vi "Msg Rescript.vi"() -> ()   [LabVIEW 2025]
uses:
  _Shared/Type.ctl
  _Shared/_Shared.lvlib
  _Msg Rescript/_Msg Rescript/_Msg Rescript.lvclass
  _Shared/Panel/Panel.lvlib
  _Shared/Tree/Tree.lvlib
  _Shared/Name Specs/Name Specs.lvclass
panel:
  out "Target":string
  in  "Tree":string(tree)
  in  "OK":bool
  # "Disclaimer: Please consider committing changes before AND after this action"
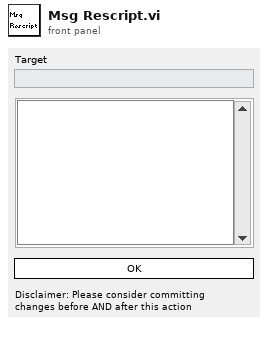
[diagram p1: front panel]
types:
  T1 = typedef "_Shared.lvlib/Type Name Library File Path.ctl" = map{T2, T3}
  T2 = typedef "_Shared.lvlib/Type.ctl" = enum16{"Actor", "Msg"}
  T3 = typedef "_Shared.lvlib/Name Library File Path.ctl" = map{string, path}
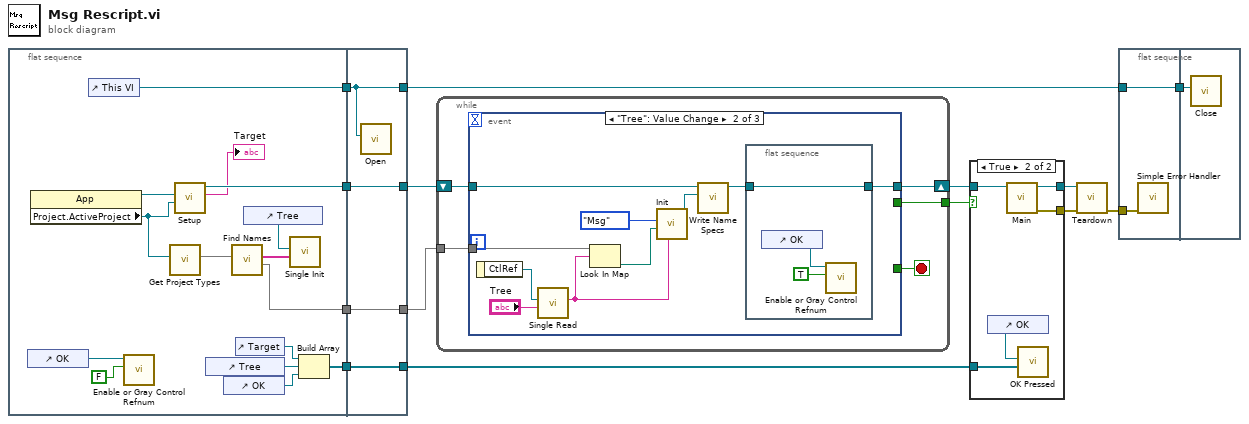
[diagram p0: block diagram]
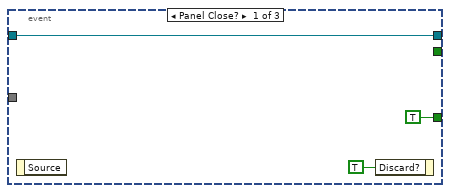
[diagram p2: hidden frame]
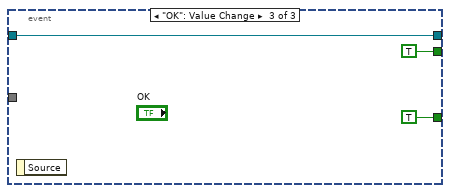
[diagram p3: hidden frame]
diagram:
  n1 = flat-sequence {
    tunnel: [w29] -> w10
    tunnel: [w18] -> w9
    tunnel: [w20] -> w6
    tunnel: [w27] -> w5
    tunnel: w10 -> [w33]
    tunnel: [w33] -> w2
    tunnel: [w32] -> w8
    tunnel: w9 -> [w32]
    tunnel: [w31] -> w7
    tunnel: w6 -> [w31]
    tunnel: [w30] -> w4
    tunnel: w5 -> [w30]
    frame #0 {
      n2 = control-ref of="OK"() -> (w26:refnum<vi>)
      n3 = property class="App"() -> (reference out=w19:refnum<vi>, "Project.ActiveProject"=w17:refnum<vi>)  [unwired: 2 in, 1 out]
      n4 = control-ref of="This VI"() -> (w29:refnum<vi>)
      n5 = call <vilib>:"Enable or Gray Control Refnum.vi"("enable?"=FALSE, "Control in"=w26) -> ()  [unwired: 8 in, 2 out]
      n6 = call "Get Project Types.vi"("Project:Active Project"=w17) -> ("Type Name Library File Path"=w21:T1)  [unwired: 10 in]
      n7 = call "Setup.vi"("Active Project"=w17, "NI.LV.Dialog Instance"=w19) -> ("Target"=→"Target":string, "_Rescript Msg out"=w18:refnum<class "_Msg Rescript.lvclass">)  [unwired: 8 in]
      n8 = control-ref of="Tree"() -> (w23:refnum<vi>)
      n9 = control-ref of="OK"() -> (w28:refnum<vi>)
      n10 = call "Find Names.vi"("Type Name Library File Path"=w21) -> ("Name Library File Path"=w20:T3, "Names"=w22:string[])  [unwired: 9 in]
      n11 = control-ref of="Target"() -> (w15:refnum<vi>)
      n12 = control-ref of="Tree"() -> (w24:refnum<vi>)
      n13 = call "Single Init.vi"("Left Cell Strings"=w22, "Tree Ref"=w24) -> ()  [unwired: 10 in]
      n14 = Build Array(w15, w23, w28) -> (w27:refnum<vi>[])
    }
    frame #1 {
      n15 = call "Open.vi"("VI"=w33) -> ()  [unwired: 11 in]
    }
  }
  n16 = while {
    tunnel: [w38] -> w12
    shift-right: [w35] -> w11
    shift-left: w8 -> [w36]
    tunnel: w7 -> [w34]
    stop <- w37 stop-if-true
    n17 = event shown="[1] \"Tree\": Value Change" {
      selector: _ -> [_ _ _]
      dyn-events: _ -> [_ _ _]
      timeout: _ -> [_ _ _]
      tunnel: [_ _ TRUE ("Rename 2")] -> w38
      tunnel: [TRUE _ TRUE] -> w37
      tunnel: w36 -> [w39 w45 w57]
      tunnel: [w39 w43 w57] -> w35
      tunnel: w34 -> [_ w51 _]
      event Panel Close? {
        n18 = event-data() -> ()  [unwired: 1 in, 1 out]
        n19 = event-data("Discard?"=TRUE) -> ()  [unwired: 1 in, 1 out]
      }
      event "Tree": Value Change {
        n20 = event-data() -> ("CtlRef"=w50:refnum<vi>)  [unwired: 1 in]
        n21 = call "Single Read.vi"("Tree"="Tree", "Tree Ref"=w50) -> ("Name"=w48:string)  [unwired: 9 in]
        n22 = Look In Map(map=w51, key=w48) -> (value=w47:path)  [unwired: 1 in, 1 out]
        n23 = call "Init.vi"("Name"=w48, "Name Library File Path"=w47, "Type"=Type."Msg") -> ("Name Specs out"=w44:refnum<class "Name Specs.lvclass">)  [unwired: 8 in]
        n24 = call "Write Name Specs.vi"("Name Specs"=w44, "_Msg Rescript in"=w45) -> ("_Msg Rescript out"=w42:refnum<class "_Msg Rescript.lvclass">)  [unwired: 9 in]
        n25 = flat-sequence {
          tunnel: [w54] -> w43
          tunnel: w42 -> [w54]
          frame #0 {
            n26 = control-ref of="OK"() -> (w53:refnum<vi>)
            n27 = call <vilib>:"Enable or Gray Control Refnum.vi"("enable?"=TRUE, "Control in"=w53) -> ()  [unwired: 8 in, 2 out]
          }
        }
      }
      event "OK": Value Change {
        n28 = event-data() -> ()  [unwired: 1 in, 1 out]
      }
    }
  }
  n29 = case shown="True" w12 {
    tunnel: w11 -> [w58 w63]
    tunnel: [w58 w62] -> w14
    tunnel: w4 -> [_ w60]
    tunnel: [_ w61] -> w13
    frame False {
    }
    frame True {
      n30 = control-ref of="OK"() -> (w59:refnum<vi>)
      n31 = call "Main.vi"("_Rescript Msg in"=w63) -> ("error out"=w61:errorcluster, "_Rescript Msg out"=w62:refnum<class "_Msg Rescript.lvclass">)  [unwired: 9 in]
      n32 = call "OK Pressed.vi"("Controls in"=w60, "OK Ref"=w59) -> ()  [unwired: 10 in]
    }
  }
  n33 = call "Teardown.vi"("error in"=w13, "_Rescript Msg in"=w14) -> ("error out"=w1:errorcluster)  [unwired: 9 in]
  n34 = flat-sequence {
    tunnel: w1 -> [w65]
    tunnel: w2 -> [w64]
    tunnel: [w64] -> w3
    tunnel: w3 -> [w66]
    frame #0 {
      n35 = call <vilib>:"Simple Error Handler.vi"("error in (no error)"=w65) -> ()  [unwired: 4 in, 5 out]
    }
    frame #1 {
      n36 = call "Close.vi"("VI"=w66) -> ()  [unwired: 11 in]
    }
  }
